vi "construct.vi"(8 "error in (no error)":errorcluster, 9 "configuration name":string, 10 "load config file?":bool=TRUE, 11 "SweepDL090926Automation in":refnum<class "SweepDL090926Automation.lvclass">) -> (0 "error out":errorcluster, 3 "SweepDL090926Automation out":refnum<class "SweepDL090926Automation.lvclass">)   [LabVIEW 2010, in "SweepDL090926Automation.lvclass"]
uses:
  SweepDL090926Automation.lvclass
  GenericSweep/GenericSweep/GenericSweep.lvclass
  ImagingMode/GenericImagingMode/GenericImagingMode/GenericImagingMode.lvclass
  SweepDL090926Automation.lvclass/SweepDL090926Automation.ctl
  common/classes/GenericComponent/GenericComponent/GenericComponent.lvclass
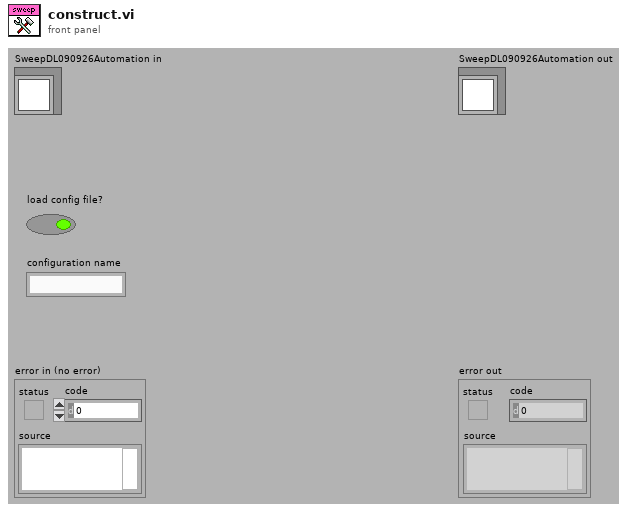
[diagram p1: front panel]
types:
  T1 = typedef "plugin_specification.ctl" = cluster{"class path":string, "configuration":string, "label":string, "settings name":string}
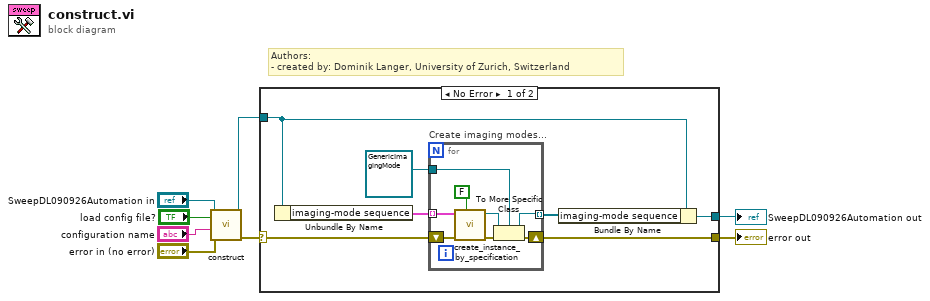
[diagram p0: block diagram]
diagram:
  # "Authors: \n- created by: Dominik Langer, University of Zurich, Switzerland"
  n1 = call-parent "construct.vi"("error in (no error)"="error in (no error)", "configuration name"="configuration name", "load config file?"="load config file?", "GenericPlugin in"="SweepDL090926Automation in") -> ("error out"=w4:errorcluster, "GenericPlugin out"=w3:refnum<class "SweepDL090926Automation.lvclass">)  [unwired: 6 in]
  n2 = case shown="No Error" w4 {
    selector: w4 -> [w14 w25]
    tunnel: w3 -> [w11 w24]
    tunnel: [w13 w25] -> w2
    tunnel: [w10 w24] -> w1
    frame No Error {
      n3 = Unbundle By Name(w11) -> ("imaging-mode sequence"=w15:T1[])
      n4 = for "Create imaging modes..." {
        tunnel: w15 -> [w21] mode=indexing
        shift-right: [w17] -> w13
        shift-left: w14 -> [w22]
        tunnel: refnum<class "GenericImagingMode.lvclass"> refnum ("GenericImagingMode.lvclass") -> [w23]
        tunnel: [w16] -> w9 mode=indexing
        n5 = call "create_instance_by_specification.vi"("call constructor?"=FALSE, "error in (no error)"=w22, "component specification"=w21) -> ("error out"=w18:errorcluster, "GenericPlugin out"=w19:refnum<class "GenericComponent.lvclass">)  [unwired: 6 in, 1 out]
        n6 = To More Specific Class(target class=w23, reference=w19, error in=w18) -> (specific class reference=w16:refnum<class "GenericImagingMode.lvclass">, error out=w17:errorcluster)
      }
      n7 = Bundle By Name(cluster=w11, "imaging-mode sequence"=w9) -> (w10:refnum<class "SweepDL090926Automation.lvclass">)
    }
    frame Error {
    }
  }
  "error out" <- w2
  "SweepDL090926Automation out" <- w1
